vi "Get_CCD_temperature.vi"(8 "error in":errorcluster, 11 "camera handle in":u64) -> (0 "error out":errorcluster, 2 "temperature(C)":dbl, 3 "camera handle out":u64)   [LabVIEW 2014, in "PICam.lvlib"]
doc: "Reads the CCD temperature in Celsius units.\nYou need to call the \"Refresh_parameters_from_camera.vi\" before reading the actual temperature, to receive the updated value from the cam to the local memory."
uses:
  PICam.lvlib
  Program Files/Princeton Instruments/PICam/Runtime/Picam32.dll
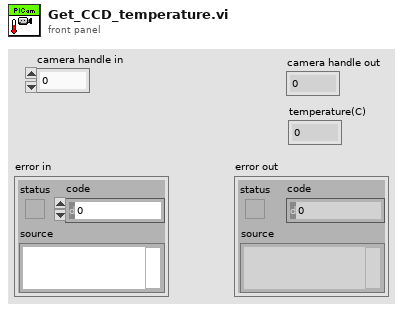
[diagram p1: front panel]
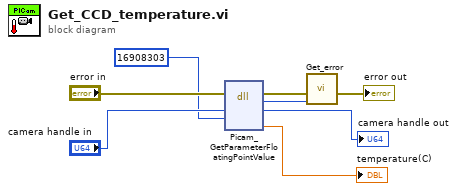
[diagram p0: block diagram]
diagram:
  n1 = dll-call lib="C:/Program Files/Princeton Instruments/PICam/Runtime/Picam32.dll" fn="Picam_GetParameterFloatingPointValue"(error in="error in", "camera"="camera handle in", "PicamParameter"=u32 16908303) -> (error out=w8:errorcluster, "return type"=w7:i32, "camera"=→"camera handle out":u64, "temperature"=→"temperature(C)":dbl)  [unwired: 4 in, 1 out]
  n2 = call "Get_error.vi"("PICam_Error"=w7, "error in (no error)"=w8) -> ("error out"=→"error out":errorcluster)  [unwired: 9 in]
